vi "onCreated.vi"(8 "error in (no error)":errorcluster, 11 "SMO.B":refnum<class "SMO.B.lvclass">) -> (0 "error out":errorcluster, 3 "SMO.B out":refnum<class "SMO.B.lvclass">)   [LabVIEW 2013, in "SMO.B.lvclass"]
uses:
  SMO.B.lvclass
  Config--cluster.ctl
  src/SMO/SMO.lvclass
panel:
  out "any found?":bool
  out "data":T1
  # "For instructions on how to use the JKI State Machine Objects, examples and video tutorials, visit:\nhttp://jki.net/state-machine-objects/\n\nJKI State Machine Objects™\nhttp://jki.net/state-machine-objects/\nCopyright (C) 2005-2015, JKI <info@jki.net>\nALL RIGHTS RESERVED"
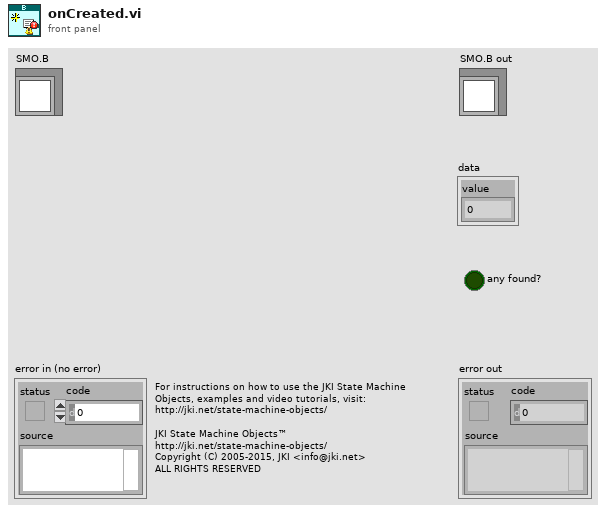
[diagram p1: front panel]
types:
  T1 = typedef "SMO.B.lvclass/Config--cluster.ctl" = cluster{"value":dbl}
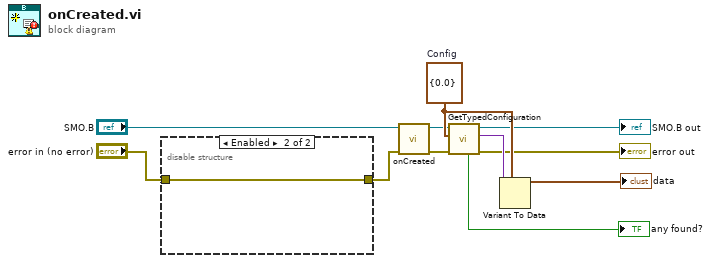
[diagram p0: block diagram]
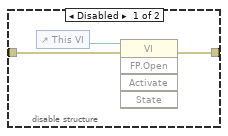
[diagram p2: hidden frame]
diagram:
  w8 = T1 {"value"=0.0}  # Config
  n1 = disable-structure shown="Enabled" {
    disable-tunnel: "error in (no error)" -> [w13 w15]
    disable-tunnel: [w12 w15] -> w1
    frame Disabled {
      n2 = control-ref of="This VI"() -> (w14:refnum<vi>)
      n3 = invoke class="VI" method="FP.Open"(reference=w14, error in=w13) -> (error out=w12:errorcluster)  [unwired: 3 in, 4 out]
    }
    frame Enabled {
    }
  }
  n4 = call-parent "onCreated.vi"("error in (no error)"=w1, "SMO"="SMO.B") -> ("error out"=w4:errorcluster, "SMO out"=w3:refnum<class "SMO.B.lvclass">)  [unwired: 8 in]
  n5 = call "GetTypedConfiguration.vi"("error in (no error)"=w4, "Default value"=w8, "SMO"=w3) -> ("error out"=→"error out":errorcluster, "Variant"=w7:variant, "SMO out"=→"SMO.B out":refnum<class "SMO.B.lvclass">, "Any Found"=→"any found?":bool)  [unwired: 4 in, 1 out]
  n6 = Variant To Data(type=w8, Variant=w7) -> (data=→"data":T1)  [unwired: 1 in, 1 out]
